vi "CAN Convert TPCANStatus_eX.vi"(11 "TPCANStatus in":u32 format="%x") -> (2 "QRCVEMPTY?":bool, 3 "TPCANStatus out":u32 format="%x", 5 "TPCANStatus-Text":string)   [LabVIEW 2017, in "PCANBasic_eX.lvlib"]
uses:
  PCANBasic_eX.lvlib
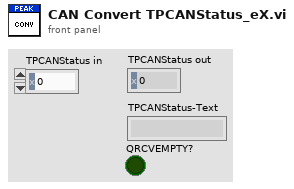
[diagram p1: front panel]
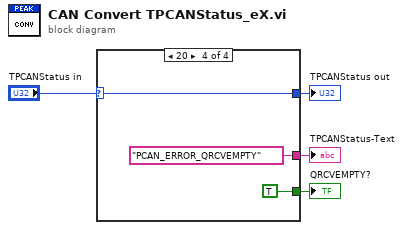
[diagram p0: block diagram]
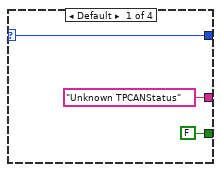
[diagram p2: hidden frame]
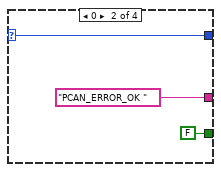
[diagram p3: hidden frame]
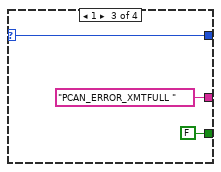
[diagram p4: hidden frame]
diagram:
  n1 = case shown="20" "TPCANStatus in" {
    selector: "TPCANStatus in" -> [w7 w9 w12 w16]
    tunnel: ["Unknown TPCANStatus" "PCAN_ERROR_OK " "PCAN_ERROR_XMTFULL " "PCAN_ERROR_QRCVEMPTY"] -> w2
    tunnel: [w7 w9 w12 w16] -> w3
    tunnel: [FALSE FALSE FALSE TRUE] -> w1
    frame Default {
    }
    frame 0 {
    }
    frame 1 {
    }
    frame 32 {
    }
  }
  "TPCANStatus out" <- w3
  "TPCANStatus-Text" <- w2
  "QRCVEMPTY?" <- w1
